vi "Edit Auton Queue Items.vi"(10 "Add?":bool, 11 "Delete?":bool) -> ()   [LabVIEW 2015]
uses:
  Robot Global Data.vi
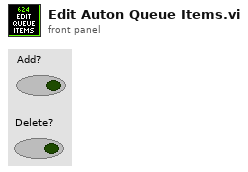
[diagram p1: front panel]
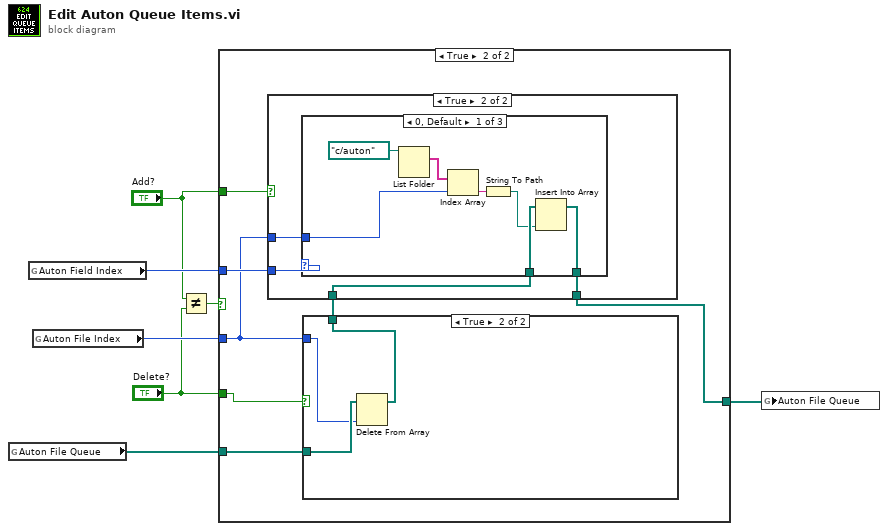
[diagram p0: block diagram]
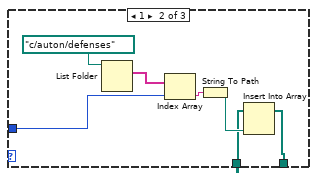
[diagram p4: hidden frame]
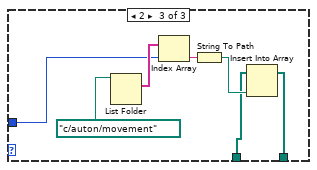
[diagram p5: hidden frame]
diagram:
  n1 = global read "Robot Global Data.vi" "Auton File Queue"() -> (w2:path[])
  n2 = global read "Robot Global Data.vi" "Auton Field Index"() -> (w7:i32)
  n3 = global read "Robot Global Data.vi" "Auton File Index"() -> (w6:i32)
  n4 = Not Equal?(x="Add?", y="Delete?") -> (x != y?=w3:bool)
  n5 = case shown="True" w3 {
    tunnel: "Add?" -> [_ w12]
    tunnel: "Delete?" -> [_ w15]
    tunnel: w7 -> [_ w11]
    tunnel: w6 -> [_ w10]
    tunnel: w2 -> [w8 w14]
    tunnel: [w8 w9] -> w1
    frame False {
    }
    frame True {
      n6 = case shown="True" w15 {
        tunnel: w10 -> [_ w44]
        tunnel: w14 -> [w42 w45]
        tunnel: [w42 w43] -> w13
        frame False {
        }
        frame True {
          n7 = Delete From Array(array=w45, index=w44) -> (array with subset deleted=w43:path[])  [unwired: 1 in, 1 out]
        }
      }
      n8 = case shown="True" w12 {
        tunnel: w13 -> [w16 w18]
        tunnel: w11 -> [_ w20]
        tunnel: w10 -> [_ w19]
        tunnel: [w16 w17] -> w9
        frame False {
        }
        frame True {
          n9 = case shown="0, Default" w20 {
            tunnel: w19 -> [w26 w30 w36]
            tunnel: w18 -> [w23 w29 w37]
            tunnel: [w21 w28 w35] -> w17
            frame 0, Default {
              n10 = List Folder(path=path "c:/auton") -> (filenames=w25:string[])  [unwired: 3 in, 3 out]
              n11 = Index Array(array=w25, index=w26) -> (element=w24:string)
              n12 = String To Path(string=w24) -> (path=w22:path)
              n13 = Insert Into Array(array=w23, new element=w22) -> (w21:path[])  [unwired: 1 in]
            }
            frame 1 {
              n14 = List Folder(path=path "c:/auton/defenses") -> (filenames=w32:string[])  [unwired: 3 in, 3 out]
              n15 = Index Array(array=w32, index=w30) -> (element=w33:string)
              n16 = String To Path(string=w33) -> (path=w34:path)
              n17 = Insert Into Array(array=w29, new element=w34) -> (w28:path[])  [unwired: 1 in]
            }
            frame 2 {
              n18 = List Folder(path=path "c:/auton/movement") -> (filenames=w39:string[])  [unwired: 3 in, 3 out]
              n19 = Index Array(array=w39, index=w36) -> (element=w40:string)
              n20 = String To Path(string=w40) -> (path=w41:path)
              n21 = Insert Into Array(array=w37, new element=w41) -> (w35:path[])  [unwired: 1 in]
            }
          }
        }
      }
    }
  }
  n22 = global write "Robot Global Data.vi" "Auton File Queue"(w1) -> ()
